vi "Configure System Tray Menu.vi"(8 "error in (no error)":errorcluster, 11 "NotifyIcon in":refnum<class "NotifyIcon.lvclass">) -> (0 "error out":errorcluster, 3 "NotifyIcon out":refnum<class "NotifyIcon.lvclass">)   [LabVIEW 2016, in "Assert API Components.lvlib" / "Assert Startup UI.lvlib" / "Assert Startup UI.lvclass"]
doc: "Builds up the menu to be used by the system tray icon tools"
uses:
  Assert Startup UI.lvclass
  System Tray/NotifyIcon.lvclass
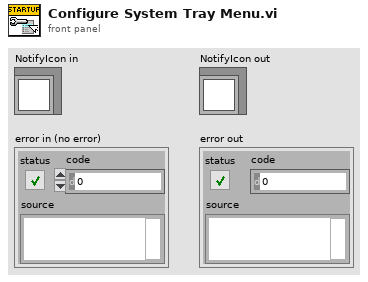
[diagram p1: front panel]
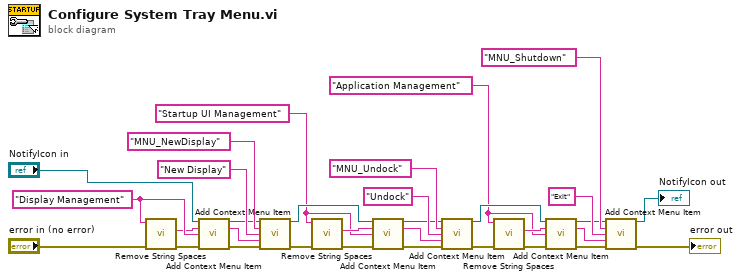
[diagram p0: block diagram]
diagram:
  w2 = "Application Management" ("Input String")
  w10 = "Startup UI Management" ("Item Tag")
  w14 = "Display Management" ("Item Text")
  n1 = call "Remove String Spaces.vi"("error in (no error)"="error in (no error)", "Input String"=w14) -> ("error out"=w15:errorcluster, "Output String"=w13:string)  [unwired: 8 in]
  n2 = call "Add Context Menu Item.vi"("NotifyIcon in"="NotifyIcon in", "Item Tag"=w13, "Item Text"=w14, "error in (no error)"=w15) -> ("NotifyIcon out"=w20:refnum<class "NotifyIcon.lvclass">, "dub Item Tag"=w9:string, "error out"=w22:errorcluster)  [unwired: 9 in]
  n3 = call "Add Context Menu Item.vi"("NotifyIcon in"=w20, "Item Tag"="MNU_NewDisplay", "Item Text"="New Display", "Parent Item Tag (\"\")"=w9, "error in (no error)"=w22) -> ("NotifyIcon out"=w18:refnum<class "NotifyIcon.lvclass">, "error out"=w25:errorcluster)  [unwired: 1 in, 8 out]
  n4 = call "Remove String Spaces.vi"("error in (no error)"=w25, "Input String"=w10) -> ("error out"=w12:errorcluster, "Output String"=w11:string)  [unwired: 8 in]
  n5 = call "Add Context Menu Item.vi"("NotifyIcon in"=w18, "Item Tag"=w11, "Item Text"=w10, "error in (no error)"=w12) -> ("NotifyIcon out"=w17:refnum<class "NotifyIcon.lvclass">, "dub Item Tag"=w8:string, "error out"=w19:errorcluster)  [unwired: 9 in]
  n6 = call "Add Context Menu Item.vi"("NotifyIcon in"=w17, "Item Tag"="MNU_Undock", "Item Text"="Undock", "Parent Item Tag (\"\")"=w8, "error in (no error)"=w19) -> ("NotifyIcon out"=w5:refnum<class "NotifyIcon.lvclass">, "error out"=w24:errorcluster)  [unwired: 1 in, 8 out]
  n7 = call "Remove String Spaces.vi"("error in (no error)"=w24, "Input String"=w2) -> ("error out"=w7:errorcluster, "Output String"=w3:string)  [unwired: 8 in]
  n8 = call "Add Context Menu Item.vi"("NotifyIcon in"=w5, "Item Tag"=w3, "Item Text"=w2, "error in (no error)"=w7) -> ("NotifyIcon out"=w4:refnum<class "NotifyIcon.lvclass">, "dub Item Tag"=w1:string, "error out"=w6:errorcluster)  [unwired: 9 in]
  n9 = call "Add Context Menu Item.vi"("NotifyIcon in"=w4, "Item Tag"="MNU_Shutdown", "Item Text"="Exit", "Parent Item Tag (\"\")"=w1, "error in (no error)"=w6) -> ("NotifyIcon out"=→"NotifyIcon out":refnum<class "NotifyIcon.lvclass">, "error out"=→"error out":errorcluster)  [unwired: 1 in, 8 out]
